vi "change_intensity_incrementally.vi"(8 "error in (no error)":errorcluster, 10 "mode":i32, 11 "ScanHeadDL090202 in":refnum<class "ScanHeadDL090202.lvclass">) -> (0 "error out":errorcluster, 3 "ScanHeadDL090202 out":refnum<class "ScanHeadDL090202.lvclass">)   [LabVIEW 2011, in "ScanHeadDL090202.lvclass"]
uses:
  ScanHeadDL090202.lvclass
  ScanHeadDL090202.lvclass/ScanHeadDL090202.ctl
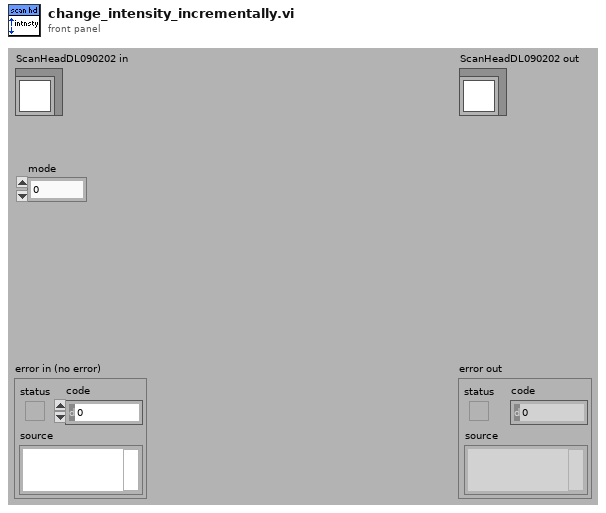
[diagram p1: front panel]
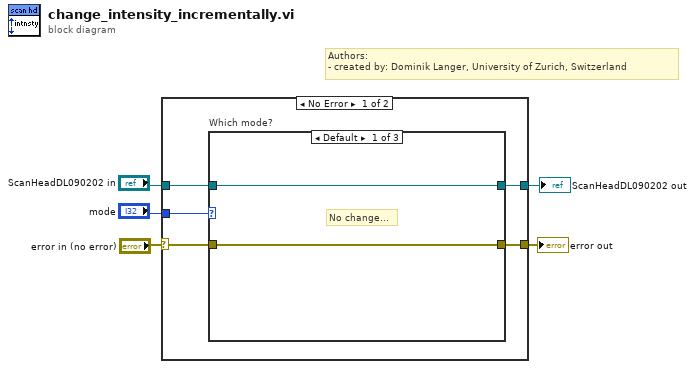
[diagram p0: block diagram]
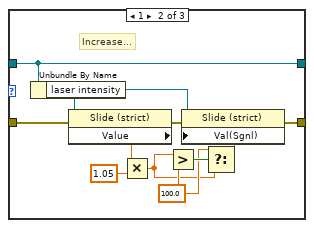
[diagram p2: hidden frame]
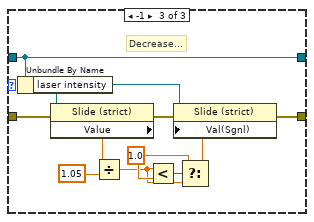
[diagram p3: hidden frame]
diagram:
  # "Authors: \n- created by: Dominik Langer, University of Zurich, Switzerland"
  n1 = case shown="No Error" "error in (no error)" {
    selector: "error in (no error)" -> [w9 w36]
    tunnel: [w10 w36] -> w4
    tunnel: [w6 w35] -> w5
    tunnel: "ScanHeadDL090202 in" -> [w7 w35]
    tunnel: "mode" -> [w8 _]
    frame No Error {
      n2 = case "Which mode?" shown="Default" w8 {
        tunnel: [w12 w20 w27] -> w10
        tunnel: w7 -> [w11 w14 w28]
        tunnel: w9 -> [w12 w19 w30]
        tunnel: [w11 w14 w28] -> w6
        frame Default {
          # "No change..."
        }
        frame 1 {
          w21 = 100.0 ("y")
          # "Increase..."
          n3 = Unbundle By Name(w14) -> ("laser intensity"=w17:refnum<vi>)
          n4 = property on="Property Node" class="Slide (strict)"(reference=w17, error in=w19) -> (error out=w18:errorcluster, "Value"=w16:dbl)  [unwired: 1 out]
          n5 = Multiply(x=w16, y=1.05) -> (x*y=w15:dbl)
          n6 = Greater?(x=w15, y=w21) -> (0:w22:bool)
          n7 = Select(t=w21, s=w22, f=w15) -> (s? t:f=w13:dbl)
          n8 = property on="Property Node" class="Slide (strict)"(reference=w17, error in=w18, "Val(Sgnl)"=w13) -> (error out=w20:errorcluster)  [unwired: 1 out]
        }
        frame -1 {
          w33 = 1.0 ("y")
          # "Decrease..."
          n9 = Unbundle By Name(w28) -> ("laser intensity"=w29:refnum<vi>)
          n10 = property on="Property Node" class="Slide (strict)"(reference=w29, error in=w30) -> (error out=w32:errorcluster, "Value"=w31:dbl)  [unwired: 1 out]
          n11 = Divide(x=w31, y=1.05) -> (x/y=w26:dbl)
          n12 = Less?(x=w26, y=w33) -> (x < y?=w34:bool)
          n13 = Select(t=w33, s=w34, f=w26) -> (s? t:f=w25:dbl)
          n14 = property on="Property Node" class="Slide (strict)"(reference=w29, error in=w32, "Val(Sgnl)"=w25) -> (error out=w27:errorcluster)  [unwired: 1 out]
        }
      }
    }
    frame Error {
    }
  }
  "error out" <- w4
  "ScanHeadDL090202 out" <- w5
